vi "Scope_decoder_8b.vi"(0 "raw_data":string) -> (1 "scope_data":T1)   [LabVIEW 2015, in "Hardware.lvlib"]
uses:
  Hardware.lvlib
  Scope data.ctl
panel:
  out "number":u8 format="%03x"
  out "LSB":dbl
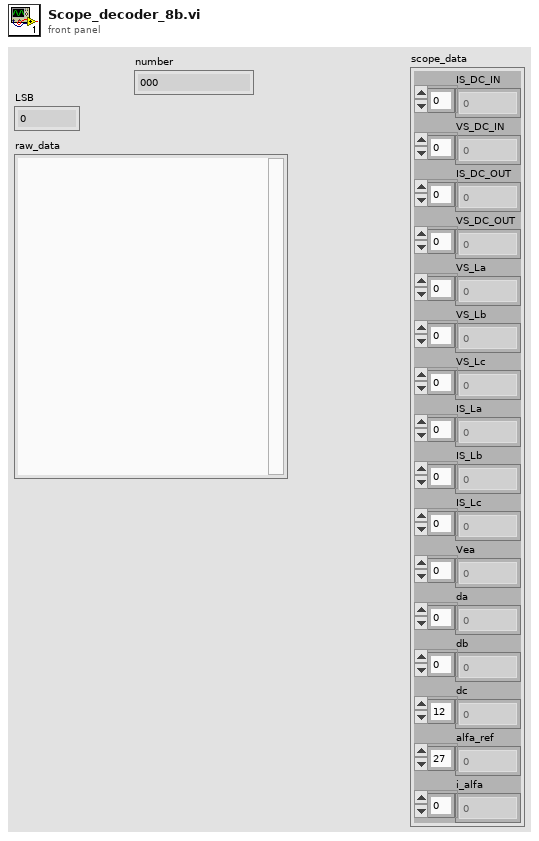
[diagram p1: front panel]
types:
  T1 = typedef "Hardware.lvlib/Scope data.ctl" = cluster{"IS_DC_IN":dbl[], "VS_DC_IN":dbl[], "IS_DC_OUT":dbl[], "VS_DC_OUT":dbl[], "VS_La":dbl[], "VS_Lb":dbl[], "VS_Lc":dbl[], "IS_La":dbl[], "IS_Lb":dbl[], "IS_Lc":dbl[], "Vea":i16[], "da":i16[], "db":i16[], "dc":i16[], "alfa_ref":dbl[], "i_alfa":dbl[]}
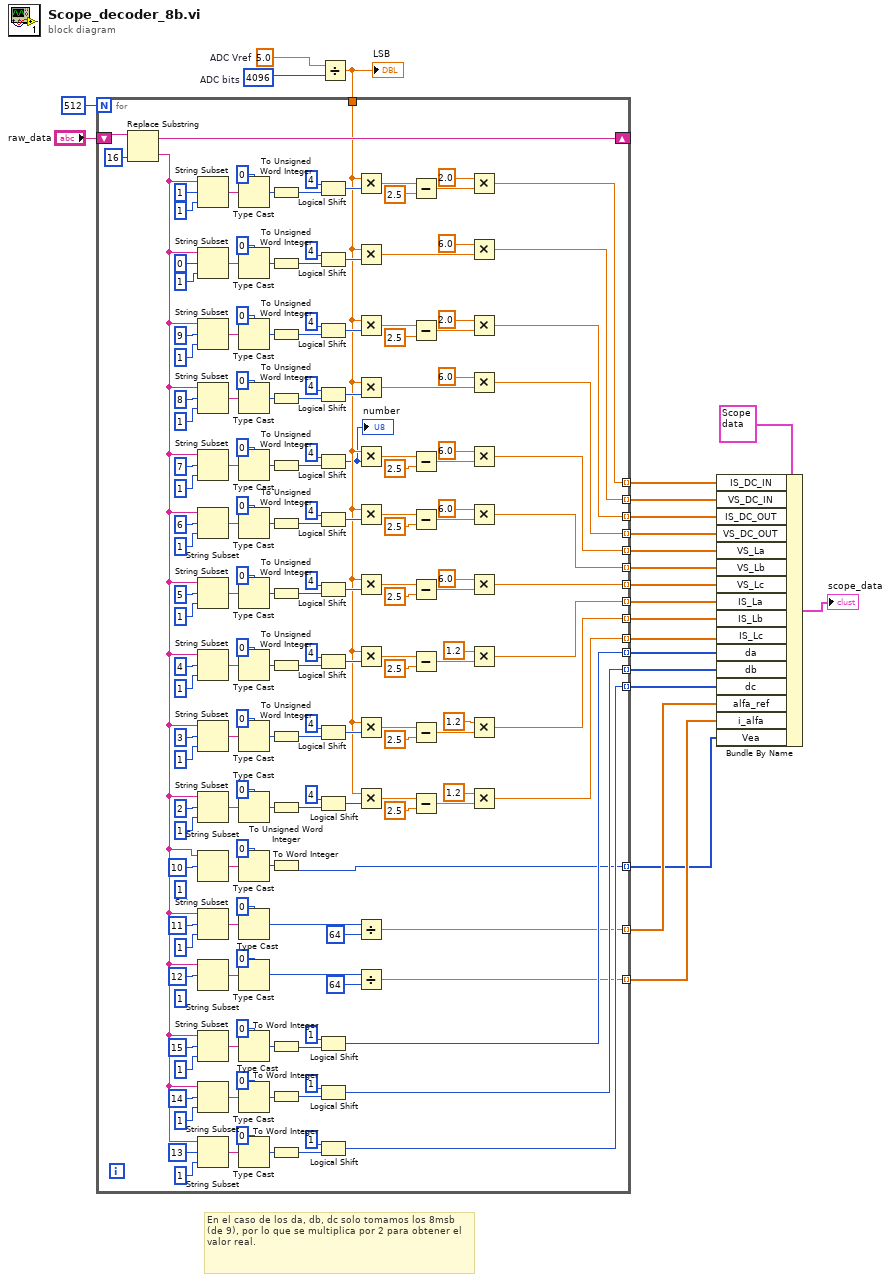
[diagram p0: block diagram]
diagram:
  w23 = 5.0  # ADC Vref
  w22 = u32 4096  # ADC bits
  # "En el caso de los da, db, dc solo tomamos los 8msb (de 9), por lo que se multiplica por 2 para obtener el valor real."
  n1 = Divide(x=w23, y=w22) -> (x/y=w19:dbl)
  "LSB" <- w19
  n2 = for {
    N: 512 -> [_]
    shift-right: [w77] -> _
    shift-left: "raw_data" -> [w78]
    tunnel: w19 -> [w66]
    tunnel: [w76] -> w18 mode=indexing
    tunnel: [w75] -> w17 mode=indexing
    tunnel: [w74] -> w16 mode=indexing
    tunnel: [w73] -> w15 mode=indexing
    tunnel: [w72] -> w14 mode=indexing
    tunnel: [w71] -> w13 mode=indexing
    tunnel: [w70] -> w12 mode=indexing
    tunnel: [w69] -> w11 mode=indexing
    tunnel: [w68] -> w10 mode=indexing
    tunnel: [w67] -> w9 mode=indexing
    tunnel: [w45] -> w8 mode=indexing
    tunnel: [w44] -> w7 mode=indexing
    tunnel: [w47] -> w6 mode=indexing
    tunnel: [w30] -> w5 mode=indexing
    tunnel: [w27] -> w4 mode=indexing
    tunnel: [w24] -> w1 mode=indexing
    (unwired) 1 ("length (rest)")
    (unwired) 1 ("length (rest)")
    n3 = Replace Substring(2:16 ("length (len. of substring)"), 5:w78) -> (0:w33:string, 1:w77:string)  [unwired: 2 in]
    n4 = String Subset(string=w33, offset (0)=1, length (rest)=1 ("length (rest)")) -> (substring=w100:string)
    n5 = String Subset(string=w33, offset (0)=0, length (rest)=1 ("length (rest)")) -> (substring=w99:string)
    n6 = String Subset(string=w33, offset (0)=9, length (rest)=1 ("length (rest)")) -> (substring=w159:string)
    n7 = String Subset(string=w33, offset (0)=8, length (rest)=1 ("length (rest)")) -> (substring=w149:string)
    n8 = String Subset(string=w33, offset (0)=7, length (rest)=1 ("length (rest)")) -> (substring=w140:string)
    n9 = String Subset(string=w33, offset (0)=6, length (rest)=1 ("length (rest)")) -> (substring=w135:string)
    n10 = String Subset(string=w33, offset (0)=5, length (rest)=1 ("length (rest)")) -> (substring=w138:string)
    n11 = String Subset(string=w33, offset (0)=4, length (rest)=1 ("length (rest)")) -> (substring=w120:string)
    n12 = String Subset(string=w33, offset (0)=3, length (rest)=1 ("length (rest)")) -> (substring=w115:string)
    n13 = String Subset(string=w33, offset (0)=2, length (rest)=1 ("length (rest)")) -> (substring=w118:string)
    n14 = String Subset(string=w33, offset (0)=10) -> (substring=w36:string)  [unwired: 1 in]
    n15 = String Subset(string=w33, offset (0)=11, length (rest)=1 ("length (rest)")) -> (substring=w38:string)
    n16 = String Subset(string=w33, offset (0)=12) -> (substring=w37:string)  [unwired: 1 in]
    n17 = String Subset(string=w33, offset (0)=15, length (rest)=1 ("length (rest)")) -> (substring=w86:string)
    n18 = String Subset(string=w33, offset (0)=14, length (rest)=1 ("length (rest)")) -> (substring=w91:string)
    n19 = String Subset(string=w33, offset (0)=13, length (rest)=1 ("length (rest)")) -> (substring=w88:string)
    n20 = Type Cast(type=u8 0 ("length (rest)"), x=w100) -> (*(type *) &x=w95:u8)
    n21 = Type Cast(type=u8 0 ("length (rest)"), x=w99) -> (*(type *) &x=w96:u8)
    n22 = Type Cast(type=u8 0 ("length (rest)"), x=w159) -> (*(type *) &x=w155:u8)
    n23 = Type Cast(type=u8 0 ("length (rest)"), x=w149) -> (*(type *) &x=w153:u8)
    n24 = Type Cast(type=u8 0 ("length (rest)"), x=w140) -> (*(type *) &x=w129:u8)
    n25 = Type Cast(type=u8 0 ("length (rest)"), x=w135) -> (*(type *) &x=w130:u8)
    n26 = Type Cast(type=u8 0 ("length (rest)"), x=w138) -> (*(type *) &x=w131:u8)
    n27 = Type Cast(type=u8 0 ("length (rest)"), x=w120) -> (*(type *) &x=w109:u8)
    n28 = Type Cast(type=u8 0 ("length (rest)"), x=w115) -> (*(type *) &x=w110:u8)
    n29 = Type Cast(type=u8 0 ("length (rest)"), x=w118) -> (*(type *) &x=w111:u8)
    n30 = Type Cast(type=i8 0 ("length (rest)"), x=w36) -> (*(type *) &x=w25:i8)
    n31 = Type Cast(type=i8 0 ("length (rest)"), x=w38) -> (*(type *) &x=w31:i8)
    n32 = Type Cast(type=i8 0 ("length (rest)"), x=w37) -> (*(type *) &x=w26:i8)
    n33 = Type Cast(type=i8 0 ("length (rest)"), x=w86) -> (*(type *) &x=w53:i8)
    n34 = Type Cast(type=i8 0 ("length (rest)"), x=w91) -> (*(type *) &x=w54:i8)
    n35 = Type Cast(type=i8 0 ("length (rest)"), x=w88) -> (*(type *) &x=w55:i8)
    n36 = To Unsigned Word Integer(number=w95) -> (unsigned 16bit integer=w65:u16)
    n37 = To Unsigned Word Integer(number=w96) -> (unsigned 16bit integer=w64:u16)
    n38 = To Unsigned Word Integer(number=w155) -> (unsigned 16bit integer=w63:u16)
    n39 = To Unsigned Word Integer(number=w153) -> (unsigned 16bit integer=w62:u16)
    n40 = To Unsigned Word Integer(number=w129) -> (unsigned 16bit integer=w61:u16)
    n41 = To Unsigned Word Integer(number=w130) -> (unsigned 16bit integer=w60:u16)
    n42 = To Unsigned Word Integer(number=w131) -> (unsigned 16bit integer=w59:u16)
    n43 = To Unsigned Word Integer(number=w109) -> (unsigned 16bit integer=w58:u16)
    n44 = To Unsigned Word Integer(number=w110) -> (unsigned 16bit integer=w57:u16)
    n45 = To Unsigned Word Integer(number=w111) -> (unsigned 16bit integer=w56:u16)
    n46 = To Word Integer(number=w25) -> (16bit integer=w24:i16)
    n47 = To Word Integer(number=w53) -> (16bit integer=w46:i16)
    n48 = To Word Integer(number=w54) -> (16bit integer=w50:i16)
    n49 = To Word Integer(number=w55) -> (16bit integer=w48:i16)
    n50 = Logical Shift(y=i16 4, x=w65) -> (x << y=w94:u16)
    n51 = Logical Shift(y=i16 4, x=w64) -> (x << y=w93:u16)
    n52 = Logical Shift(y=i16 4, x=w63) -> (x << y=w154:u16)
    n53 = Logical Shift(y=i16 4, x=w62) -> (x << y=w147:u16)
    n54 = Logical Shift(y=i16 4, x=w61) -> (x << y=w32:u16)
    "number" <- w32
    n55 = Logical Shift(y=i16 4, x=w60) -> (x << y=w128:u16)
    n56 = Logical Shift(y=i16 4, x=w59) -> (x << y=w127:u16)
    n57 = Logical Shift(y=i16 4, x=w58) -> (x << y=w108:u16)
    n58 = Logical Shift(y=i16 4, x=w57) -> (x << y=w107:u16)
    n59 = Logical Shift(y=i16 4, x=w56) -> (x << y=w106:u16)
    n60 = Logical Shift(y=i16 1, x=w46) -> (x << y=w45:i16)
    n61 = Logical Shift(y=i16 1, x=w50) -> (x << y=w44:i16)
    n62 = Logical Shift(y=i16 1, x=w48) -> (x << y=w47:i16)
    n63 = Multiply(x=w66, y=w94) -> (x*y=w186:dbl)
    n64 = Multiply(x=w66, y=w93) -> (x*y=w188:dbl)
    n65 = Multiply(x=w66, y=w154) -> (x*y=w195:dbl)
    n66 = Multiply(x=w66, y=w147) -> (x*y=w193:dbl)
    n67 = Multiply(x=w66, y=w32) -> (x*y=w182:dbl)
    n68 = Multiply(x=w66, y=w128) -> (x*y=w179:dbl)
    n69 = Multiply(x=w66, y=w127) -> (x*y=w174:dbl)
    n70 = Multiply(x=w66, y=w108) -> (x*y=w163:dbl)
    n71 = Multiply(x=w66, y=w107) -> (x*y=w166:dbl)
    n72 = Multiply(x=w66, y=w106) -> (x*y=w171:dbl)
    n73 = Divide(x=w31, y=i8 64 ("x")) -> (x/y=w30:dbl)
    n74 = Divide(x=w26, y=64 ("x")) -> (x/y=w27:dbl)
    n75 = Subtract(x=w186, y=2.5 ("x")) -> (x-y=w190:dbl)
    n76 = Subtract(x=w195, y=2.5 ("x")) -> (x-y=w191:dbl)
    n77 = Subtract(x=w182, y=2.5 ("x")) -> (x-y=w184:dbl)
    n78 = Subtract(x=w179, y=2.5 ("x")) -> (x-y=w177:dbl)
    n79 = Subtract(x=w174, y=2.5 ("x")) -> (x-y=w176:dbl)
    n80 = Subtract(x=w163, y=2.5 ("x")) -> (x-y=w161:dbl)
    n81 = Subtract(x=w166, y=2.5 ("x")) -> (x-y=w168:dbl)
    n82 = Subtract(x=w171, y=2.5 ("x")) -> (x-y=w169:dbl)
    n83 = Multiply(x=2.0, y=w190) -> (x*y=w76:dbl)
    n84 = Multiply(x=6.0, y=w188) -> (x*y=w75:dbl)
    n85 = Multiply(x=2.0, y=w191) -> (x*y=w74:dbl)
    n86 = Multiply(x=6.0, y=w193) -> (x*y=w73:dbl)
    n87 = Multiply(x=6.0, y=w184) -> (x*y=w72:dbl)
    n88 = Multiply(x=6.0, y=w177) -> (x*y=w71:dbl)
    n89 = Multiply(x=6.0, y=w176) -> (x*y=w70:dbl)
    n90 = Multiply(x=1.2, y=w161) -> (x*y=w69:dbl)
    n91 = Multiply(x=1.2, y=w168) -> (x*y=w68:dbl)
    n92 = Multiply(x=1.2, y=w169) -> (x*y=w67:dbl)
  }
  n93 = Bundle By Name(cluster=T1 {"IS_DC_IN"=[], "VS_DC_IN"=[], "IS_DC_OUT"=[], "VS_DC_OUT"=[], "VS_La"=[], "VS_Lb"=[], "VS_Lc"=[], "IS_La"=[], "IS_Lb"=[], "IS_Lc"=[], "Vea"=[], "da"=[], "db"=[], "dc"=[], "alfa_ref"=[], "i_alfa"=[]} ("scope_data"), "IS_DC_IN"=w18, "VS_DC_IN"=w17, "IS_DC_OUT"=w16, "VS_DC_OUT"=w15, "VS_La"=w14, "VS_Lb"=w13, "VS_Lc"=w12, "IS_La"=w11, "IS_Lb"=w10, "IS_Lc"=w9, "da"=w8, "db"=w7, "dc"=w6, "alfa_ref"=w5, "i_alfa"=w4, "Vea"=w1) -> (→"scope_data":T1)
